vi "Close Instrument.vi"(7 "Go Local (\"@LOC\")":bool=TRUE, 8 "error in (no error)":errorcluster, 11 "VNA-ZNB in":refnum<class "VNA-ZNB.lvclass">) -> (0 "error out":errorcluster, 3 "VNA-ZNB out":refnum<class "VNA-ZNB.lvclass">)   [LabVIEW 2020, in "VNA-ZNB.lvclass"]
uses:
  VNA-ZNB.lvclass
  C:/Sandbox/Git_Sandbox/WiSpry Test Framework source code (LV20)/WiSpry Test Framework/Instruments/Instrument.lvclass
  Instrument.lvclass/Instrument.ctl
  Vector Network Analyzer.lvclass
  Instrument.lvclass
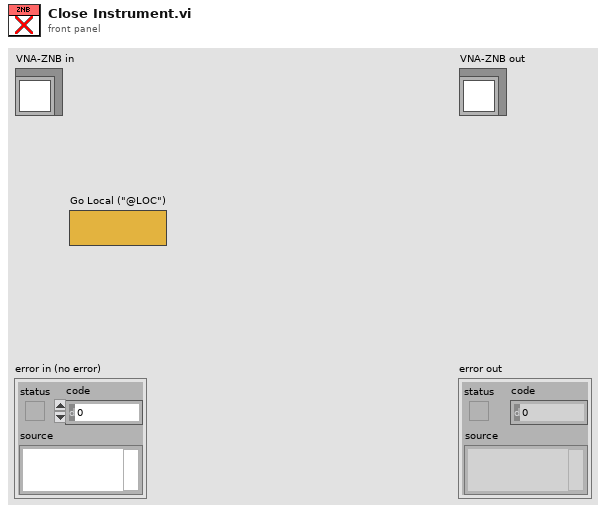
[diagram p1: front panel]
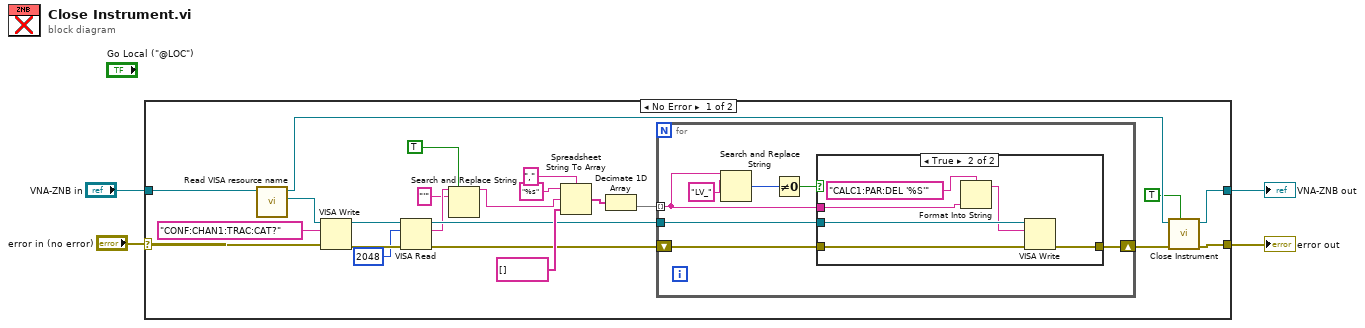
[diagram p0: block diagram]
diagram:
  n1 = case shown="No Error" "error in (no error)" {
    selector: "error in (no error)" -> [w26 w42]
    tunnel: "VNA-ZNB in" -> [w27 w43]
    tunnel: [w11 w42] -> w2
    tunnel: [w10 w43] -> w1
    frame No Error {
      n2 = call "Read VISA resource name.vi"("Instrument in"=w27) -> ("VISA resource name"=w25:refnum<visa-resource-name>, "Instrument out"=w12:refnum<class "VNA-ZNB.lvclass">)  [unwired: 9 in]
      n3 = VISA Write(VISA resource name=w25, write buffer="CONF:CHAN1:TRAC:CAT?", error in (no error)=w26) -> (VISA resource name out=w22:refnum<visa-resource-name>, error out=w23:errorcluster)  [unwired: 1 out]
      n4 = VISA Read(VISA resource name=w22, byte count=u32 2048, error in (no error)=w23) -> (VISA resource name out=w16:refnum<visa-resource-name>, read buffer=w9:string, error out=w15:errorcluster)  [unwired: 1 out]
      n5 = Search and Replace String(replace all?=TRUE ("replace all? (F)"), input string=w9, search string="'") -> (result string=w7:string)  [unwired: 5 in, 3 out]
      n6 = Spreadsheet String To Array(delimiter (Tab)=",", format string="%s", spreadsheet string=w7, array type (2D Dbl)=string[] []) -> (array=w17:string[])
      n7 = Decimate 1D Array(w17) -> (w14:string[])  [unwired: 1 out]
      n8 = for {
        tunnel: w16 -> [w31]
        shift-right: [w28] -> w13
        shift-left: w15 -> [w30]
        tunnel: w14 -> [w29] mode=indexing
        n9 = Search and Replace String(input string=w29, search string="LV_") -> (number of replacements=w33:i32)  [unwired: 6 in, 3 out]
        n10 = Not Equal To 0?(x=w33) -> (x != 0?=w32:bool)
        n11 = case shown="True" w32 {
          tunnel: w31 -> [_ w40]
          tunnel: w30 -> [w35 w39]
          tunnel: w29 -> [_ w41]
          tunnel: [w35 w38] -> w28
          frame False {
          }
          frame True {
            n12 = Format Into String(format string="CALC1:PAR:DEL '%S'" ("string"), w41) -> (resulting string=w36:string)  [unwired: 2 in, 1 out]
            n13 = VISA Write(VISA resource name=w40, write buffer=w36, error in (no error)=w39) -> (error out=w38:errorcluster)  [unwired: 2 out]
          }
        }
      }
      n14 = call-parent "Close Instrument.vi"("Go Local (\"@LOC\")"=TRUE ("Go Local (\"@LOC\")"), "error in (no error)"=w13, "Instrument in"=w12) -> ("error out"=w11:errorcluster, "Instrument out"=w10:refnum<class "VNA-ZNB.lvclass">)  [unwired: 7 in]
    }
    frame Error {
    }
  }
  "error out" <- w2
  "VNA-ZNB out" <- w1
